vi "finish5RobotsKeeperGame.vi"(8 "error in (no error)":errorcluster, 9 "Game":refnum<class "Game.lvclass">, 10 "command_interpreted":T1, 11 "5RobotsKeeperGame in":refnum<class "5RobotsKeeperGame.lvclass">) -> (0 "error out":errorcluster, 2 "finish?":bool, 3 "5RobotsKeeperGame out":refnum<class "5RobotsKeeperGame.lvclass">)   [LabVIEW 2021, in "5RobotsKeeperGame.lvclass"]
uses:
  5RobotsKeeperGame.lvclass
  Referee_class/command_interpreted.ctl
  Game_class/Game.lvclass
  Utilities_class/Utilities.lvclass
  Game_class/Game.lvclass/Game.ctl
  Ball_class/Ball.lvclass/Ball.ctl
  Team_class/Team.lvclass/Team.ctl
  Parameters_class/Parameters.lvclass/Parameters.ctl
  Game_class/Read Parameters.lvclass.vi
  Parameters_class/Read BallVelToAbortPass.vi
  Game_class/Read BallRef.vi
  Game_class/Read KeeperTeam.vi
  Team_class/Read RobotRef.vi
  Ball_class/Read v_x.vi
  Ball_class/Read v_y.vi
  Ally_class/Ally.lvclass
  D:/RoboIme/horie/SSL_AI/Team_class/Team.lvclass
  Ball_class/Ball.lvclass
  Robot_class/Robot.lvclass
  Parameters_class/Parameters.lvclass
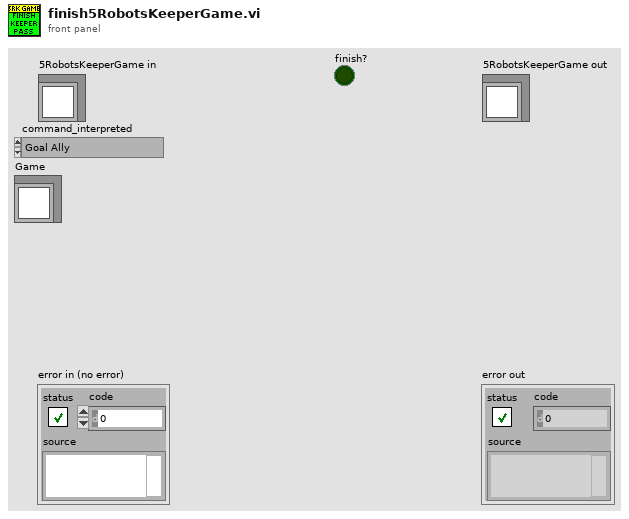
[diagram p1: front panel]
types:
  T1 = typedef "command_interpreted.ctl" = enum16{"Goal Ally", "Goal Enemy", "Ball Placement Enemy", "Ball Placement Ally", "Normal Half Time", "Extra Time  Break", "Extra Half Time", "None", "Post Game", "PKA Normal Start", "Prepare Kickoff Ally", "PKE Normal Start", "Prepare Kickoff Enemy", "Force Start", "Halt", "Timeout", "Prepare Penalty Ally", "Prepare Penalty Enemy", "PPA NormalStart", "PPE Normal Start", "Indirect Free Ally", "Direct Free Enemy", "Direct Free Ally", "Indirect Free Enemy", "Stop"}
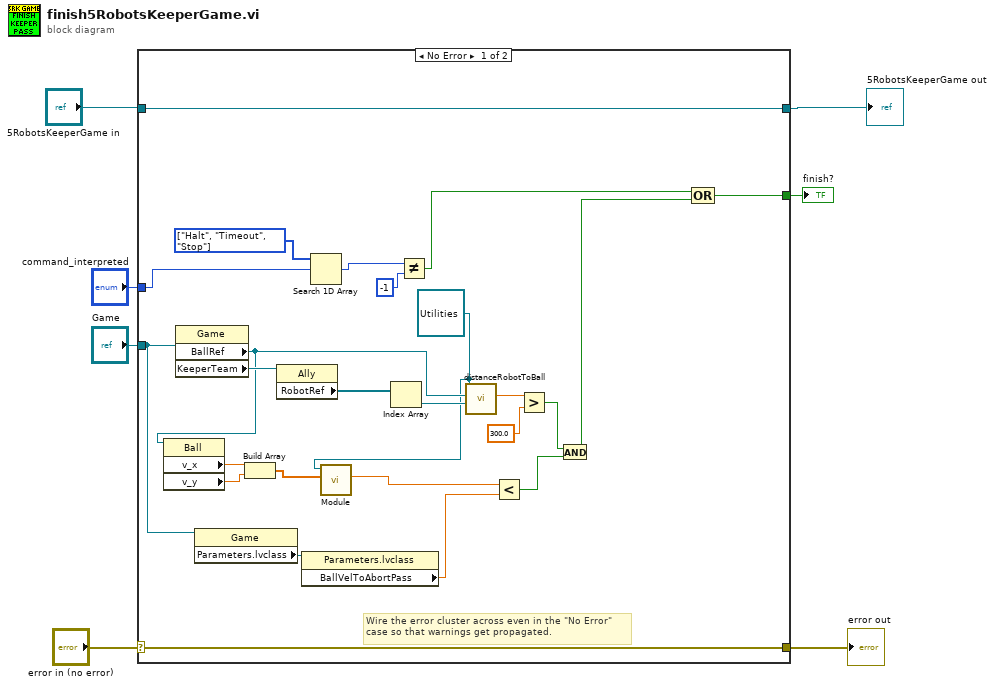
[diagram p0: block diagram]
diagram:
  n1 = case shown="No Error" "error in (no error)" {
    selector: "error in (no error)" -> [w31 w34]
    tunnel: [w31 w34] -> w7
    tunnel: [w32 w33] -> w4
    tunnel: "5RobotsKeeperGame in" -> [w32 w33]
    tunnel: "command_interpreted" -> [w29 _]
    tunnel: [w8 _] -> w3
    tunnel: "Game" -> [w9 _]
    frame No Error {
      w15 = refnum<class "Utilities.lvclass"> refnum ("Utilities in")
      w30 = T1[] [enum."Halt", enum."Timeout", enum."Stop"] items=["Goal Ally", "Goal Enemy", "Ball Placement Enemy", "Ball Placement Ally", "Normal Half Time", "Extra Time  Break", "Extra Half Time", "None", "Post Game", "PKA Normal Start", "Prepare Kickoff Ally", "PKE Normal Start", "Prepare Kickoff Enemy", "Force Start", "Halt", "Timeout", "Prepare Penalty Ally", "Prepare Penalty Enemy", "PPA NormalStart", "PPE Normal Start", "Indirect Free Ally", "Direct Free Enemy", "Direct Free Ally", "Indirect Free Enemy", "Stop"] ("Array")
      # "Wire the error cluster across even in the \"No Error\"\ncase so that warnings get propagated."
      n2 = property class="Game"(reference=w9) -> ("BallRef"=w19:refnum<class "Ball.lvclass">, "KeeperTeam"=w25:refnum<class "Ally.lvclass">)  [unwired: 1 in, 2 out]
      n3 = property class="Ball"(reference=w19) -> ("v_x"=w18:dbl, "v_y"=w17:dbl)  [unwired: 1 in, 2 out]
      n4 = property class="Game"(reference=w9) -> ("Parameters.lvclass"=w11:refnum<class "Parameters.lvclass">)  [unwired: 1 in, 2 out]
      n5 = Build Array(w18, w17) -> (w16:dbl[])
      n6 = property class="Ally"(reference=w25) -> ("RobotRef"=w24:refnum<class "Robot.lvclass">[])  [unwired: 1 in, 2 out]
      n7 = property class="Parameters.lvclass"(reference=w11) -> ("BallVelToAbortPass"=w10:dbl)  [unwired: 1 in, 2 out]
      n8 = Search 1D Array(1D array=w30, element=w29) -> (index of element=w28:i32)  [unwired: 1 in]
      n9 = call "Module.vi"("2D vector"=w16, "Utilities in"=w15) -> ("Modulo"=w20:dbl)  [unwired: 7 in, 2 out]
      n10 = Index Array(array=w24) -> (element=w23:refnum<class "Robot.lvclass">)  [unwired: 1 in]
      n11 = Not Equal?(x=w28, y=-1) -> (x != y?=w26:bool)
      n12 = call "distanceRobotToBall.vi"("Robot"=w23, "Ball"=w19, "Utilities in"=w15) -> ("Distance Robot To Ball"=w21:dbl)  [unwired: 6 in, 2 out]
      n13 = Less?(x=w20, y=w10) -> (x < y?=w14:bool)
      n14 = Greater?(x=w21, y=300.0) -> (0:w13:bool)
      n15 = And(x=w13, y=w14) -> (x .and. y?=w12:bool)
      n16 = Compound Arithmetic op=OR(w26, w12) -> (w8:bool)
    }
    frame Error {
    }
  }
  "error out" <- w7
  "5RobotsKeeperGame out" <- w4
  "finish?" <- w3
